vi "FGV reentrant.vi"(8 "Error In":errorcluster, 9 "Data":variant, 10 "Attribute Name":string, 11 "Action (read)":T1(ring)=enum."read") -> (0 "Error Out":errorcluster, 1 "Data":variant, 2 "Success":bool, 4 "Attributes":string[](array[string]), 6 "values":variant[](array[variant]))   [LabVIEW 2012, in "CS++Base.lvlib"]
doc: "This is a reentrant FGV using variant attributes to staore data. The lookup time is O(log(n)).\n\n<B>Attention:</B> This reentrant FGV must be wrapped into a non-reentrant VI for a specific database."
uses:
  CS++Base.lvlib
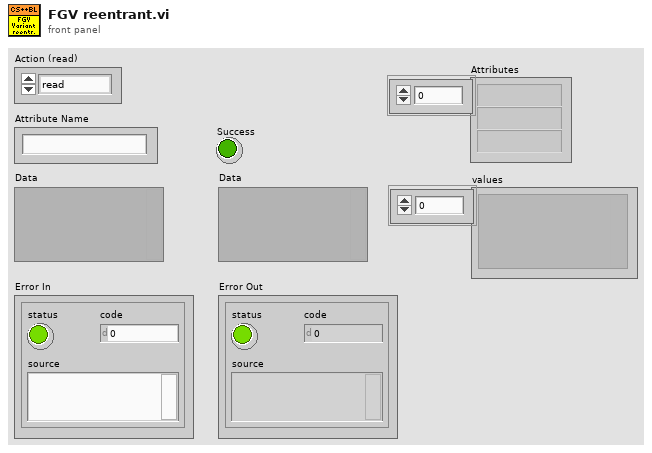
[diagram p1: front panel]
types:
  T1 = enum16{"add", "replace", "read", "remove", "reset", "get attibutes", ""}
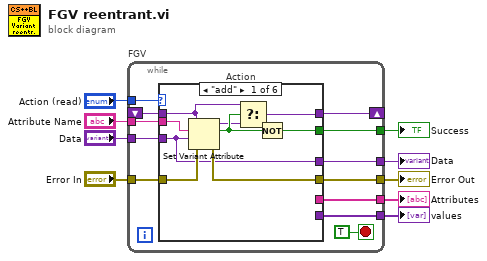
[diagram p0: block diagram]
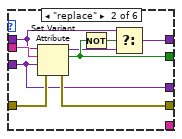
[diagram p2: hidden frame]
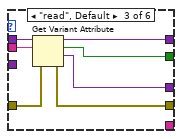
[diagram p3: hidden frame]
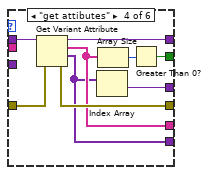
[diagram p4: hidden frame]
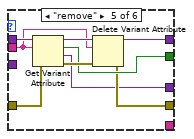
[diagram p5: hidden frame]
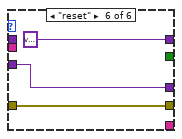
[diagram p6: hidden frame]
diagram:
  n1 = while "FGV" {
    tunnel: "Action (read)" -> [w20]
    shift-right: [w19] -> _
    shift-left: _ -> [w18]
    tunnel: "Attribute Name" -> [w17]
    tunnel: "Data" -> [w16]
    tunnel: "Error In" -> [w15]
    tunnel: [w14] -> w5
    tunnel: [w13] -> w4
    tunnel: [w12] -> w3
    tunnel: [w11] -> w2
    tunnel: [w10] -> w1
    stop <- TRUE stop-if-true
    n2 = case "Action" shown="\"add\"" w20 {
      tunnel: [w23 w33 w43 w54 w64 variant] -> w19
      tunnel: w18 -> [w25 w34 w46 w55 w62 _]
      tunnel: w17 -> [w30 w39 w45 _ w60 _]
      tunnel: w16 -> [w27 w36 _ _ _ w65]
      tunnel: w15 -> [w29 w38 w44 w53 w58 w66]
      tunnel: [w27 w36 w42 w48 w56 w65] -> w14
      tunnel: [w28 w37 w41 w52 w57 w66] -> w13
      tunnel: [w22 w35 w40 w47 w59 _] -> w12
      tunnel: [_ _ _ w51 _ _] -> w11
      tunnel: [_ _ _ w49 _ _] -> w10
      frame "add" {
        n3 = Set Variant Attribute(Variant=w25, name=w30, value=w27, error in=w29) -> (Variant out=w24:variant, replaced=w26:bool, error out=w28:errorcluster)
        n4 = Select(t=w25, s=w26, f=w24) -> (s? t:f=w23:variant)
        n5 = Not(x=w26) -> (.not. x?=w22:bool)
      }
      frame "replace" {
        n6 = Set Variant Attribute(Variant=w34, name=w39, value=w36, error in=w38) -> (Variant out=w32:variant, replaced=w35:bool, error out=w37:errorcluster)
        n7 = Not(x=w35) -> (.not. x?=w31:bool)
        n8 = Select(t=w34, s=w31, f=w32) -> (s? t:f=w33:variant)
      }
      frame "read", Default {
        n9 = Get Variant Attribute(Variant=w46, name=w45, error in=w44) -> (duplicate Variant=w43:variant, found=w40:bool, value=w42:variant, error out=w41:errorcluster)  [unwired: 1 in]
      }
      frame "get attibutes" {
        n10 = Get Variant Attribute(Variant=w55, error in=w53) -> (duplicate Variant=w54:variant, names=w51:string[], values=w49:variant[], error out=w52:errorcluster)  [unwired: 2 in]
        n11 = Index Array(array=w49) -> (element=w48:variant)  [unwired: 1 in]
        n12 = Array Size(array=w51) -> (size(s)=w50:i32)
        n13 = Greater Than 0?(x=w50) -> (x > 0?=w47:bool)
      }
      frame "remove" {
        n14 = Get Variant Attribute(Variant=w62, name=w60, error in=w58) -> (duplicate Variant=w61:variant, found=w59:bool, value=w56:variant, error out=w63:errorcluster)  [unwired: 1 in]
        n15 = Delete Variant Attribute(4:w63, 6:w60, 7:w61) -> (0:w57:errorcluster, 3:w64:variant)  [unwired: 1 out]
      }
      frame "reset" {
      }
    }
  }
  "Error Out" <- w4
  "Data" <- w5
  "Success" <- w3
  "values" <- w1
  "Attributes" <- w2
